vi "Write Pot.vi"(8 "error in (no error)":errorcluster, 10 "Pot Value(0-127)":u8, 11 "MCP4018 Digipot in":refnum<class "MCP4018 Digipot.lvclass">) -> (0 "error out":errorcluster, 3 "MCP4018 Digipot out":refnum<class "MCP4018 Digipot.lvclass">)   [LabVIEW 2020, in "CTI-Peripheral.lvlib" / "MCP4018 Digipot.lvclass"]
uses:
  MCP4018 Digipot.lvclass/MCP4018 Digipot.ctl
  CTI/I2C Connection/I2C Connection.lvclass/I2C Connection.ctl
  MCP4018 Digipot.lvclass
  CTI/I2C Connection/I2C Connection.lvclass
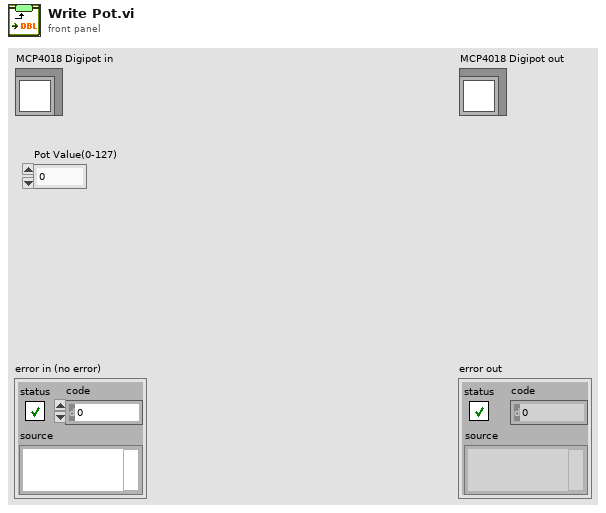
[diagram p1: front panel]
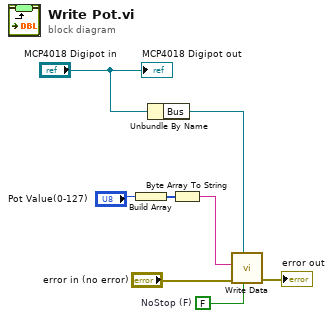
[diagram p0: block diagram]
diagram:
  w5 = FALSE  # NoStop (F)
  n1 = Build Array("Pot Value(0-127)") -> (w1:u8[])
  n2 = Unbundle By Name("MCP4018 Digipot in") -> ("Bus"=w6:refnum<class "I2C Connection.lvclass">)
  n3 = Byte Array To String(unsigned byte array=w1) -> (string=w3:string)
  n4 = call "Write Data.vi"("NoStop (F)"=w5, "I2C Connection"=w6, "error in (no error)"="error in (no error)", "Data"=w3) -> ("error out"=→"error out":errorcluster)  [unwired: 7 in]
  "MCP4018 Digipot out" <- "MCP4018 Digipot in"
